vi "Set Read Index.vi"(0 "TDMS In":refnum<k34>, 5 "Read_Index(0)":i64, 9 "Enable(True)":bool=TRUE, 11 "Error In":errorcluster) -> (4 "TDMS Out":refnum<k34>, 15 "Error Out":errorcluster)   [LabVIEW 2015, in "Teaching File.lvlib"]
doc: "Set value to the <b>Read_Index</b> property in the TDMS file."
uses:
  Teaching File.lvlib
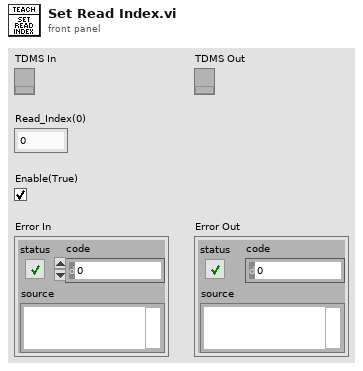
[diagram p1: front panel]
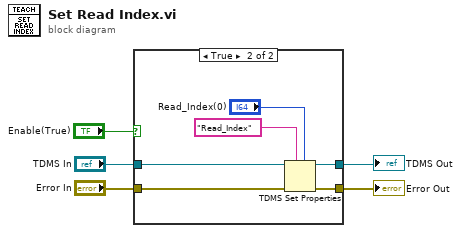
[diagram p0: block diagram]
diagram:
  n1 = case shown="True" "Enable(True)" {
    tunnel: [w7 w13] -> w5
    tunnel: [w6 w12] -> w4
    tunnel: "TDMS In" -> [w7 w11]
    tunnel: "Error In" -> [w6 w10]
    frame False {
    }
    frame True {
      n2 = TDMS Set Properties(5:"Read_Index(0)", 7:"Read_Index" ("property name"), 8:w10, 11:w11) -> (0:w12:errorcluster, 3:w13:refnum<k34>)  [unwired: 2 in, 2 out]
    }
  }
  "TDMS Out" <- w5
  "Error Out" <- w4
